vi "TEST_bench_Hyst_op_fxp_16_5.vi"(7 "N_hyst":i32) -> ()   [LabVIEW 2017]
uses:
  <vilib>/Platform/TimedLoop/XDataNode/timing_clust.ctl
  <vilib>/Platform/TimedLoop/XDataNode/nitl_modes.ctl
  <vilib>/Platform/TimedLoop/XDataNode/wakeup.ctl
  <vilib>/rvi/Emulation/niFpgaSctlEmulationGetInTimedLoop.vi
  <vilib>/rvi/Emulation/niFpgaEmulationReportErrorSimple.vi
  <vilib>/rvi/Emulation/niFpgaGetClockAttributes.vi
  <vilib>/rvi/Emulation/niFpgaCriticalErrorInLSC.vi
  <vilib>/rvi/Memory/Memory_Emulation/nirvimemoryFastEmulation.vi
  <vilib>/rvi/Memory/Memory_Emulation/nirvimemoryEmulation.vi
  <vilib>/rvi/Emulation/niFpgaEmulationIsFPGAContextNoSignature.vi
  <vilib>/rvi/DataTransferAndStorage/Container/Common/niFpgaContainerGetUniqueNameForEmu.vi
  <vilib>/rvi/Emulation/niFpgaProcessEmulError.vi
  <vilib>/rvi/errors/nirviReportUnexpectedCaseInternalError (U32).vi
  <vilib>/Platform/TimedLoop/XDataNode/XDataNode.xnode
  <vilib>/rvi/DataTransferAndStorage/Container/XNode/niFpgaContainer.xnode
  <vilib>/Platform/TimedLoop/XDataNode/XDNodeRunTimeDep.lvlib
panel:
  out "y_out_mem":fxp<+/-,16,5>[](array[numeric])
  out "S_of_ik (expected)":sgl[](array[numeric])
  out "H_of_uk":fxp<+/-,32,10>[](array[numeric])
  in  "uk":sgl[](array[numeric]) format="%#_13g"
  in  "numIter":i32
  in  "r_s":fxp<+/-,16,5>[](array[numeric])=[0.0, 0.82861328125, 1.8125, 2.8671875, 4.03173828125, 5.2001953125, 7.20166015625]
  in  "w_s":fxp<+/-,16,5>[](array[numeric])=[0.0, 0.0, 0.0, 0.0, 0.0, 0.0, 0.0]
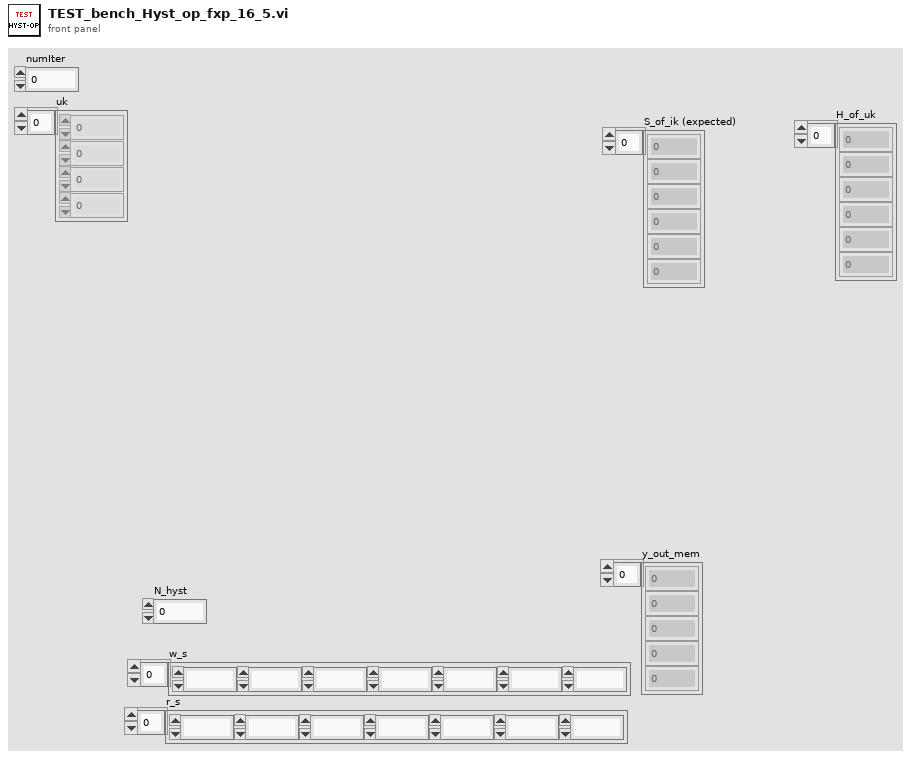
[diagram p1: front panel]
types:
  T1 = typedef "XDNodeRunTimeDep.lvlib/timing_clust.ctl" = cluster{"Expected End [f-1]":u64, "Actual End [f-1]":u64, "Finished Late? [f-1]":bool, "Expected End [i-1]":u64, "Actual End [i-1]":u64, "Finished Late? [i-1]":bool, "Expected Start [i]":u64, "Actual Start [i]":u64, "Expected Start [f]":u64, "Actual Start [f]":u64, "Source Name":string, "Structure Name":string, "Period":i64, "Deadline":i64, "Offset":i64, "Start":i64, "Priority":i32, "Timeout":i32, "Mode":T2, "Wakeup Reason":T3, "Error":errorcluster, "Source Type":string, "Secondary Source Type":string, "Global End Time":u64, "Global Start Time":u64, "Frame Duration":u64, "Iteration Duration":u64, "Assigned CPU":i32, "I/O Scan Engine Mode":u32}
  T2 = typedef "XDNodeRunTimeDep.lvlib/nitl_modes.ctl" = enum32{"No Change", "Process missed periods, maintain original phase", "Discard missed periods, maintain original phase", "Process missed periods, ignore original phase", "Discard missed periods, ignore original phase"}
  T3 = typedef "XDNodeRunTimeDep.lvlib/wakeup.ctl" = enum32{"Normal", "Aborted", "Asynchronous wakeup", "Timing source error", "Timed loop error", "Timeout"}
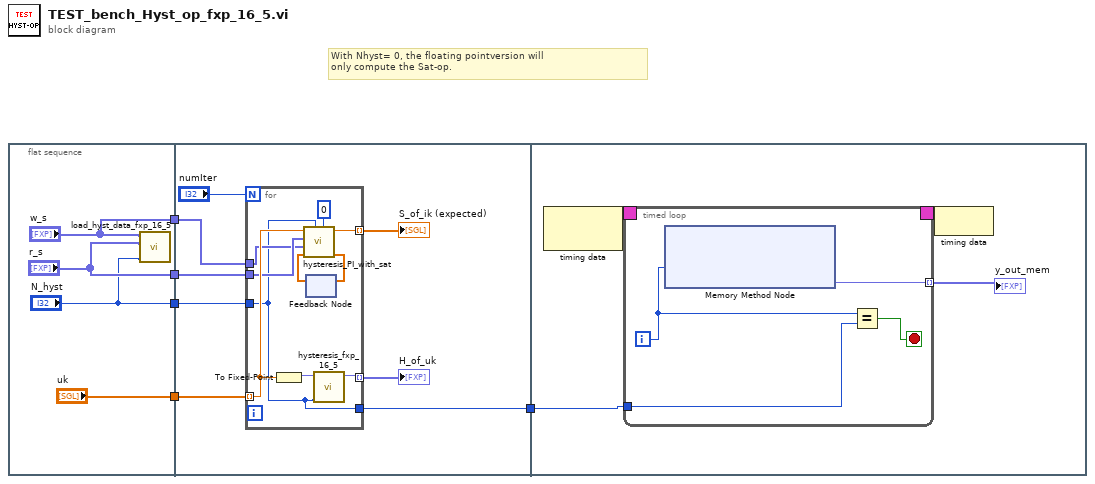
[diagram p0: block diagram]
diagram:
  # "With Nhyst= 0, the floating pointversion will\nonly compute the Sat-op."
  n1 = flat-sequence {
    tunnel: ["uk"] -> w5
    tunnel: ["w_s"] -> w4
    tunnel: ["r_s"] -> w3
    tunnel: ["N_hyst"] -> w2
    tunnel: w5 -> [w14]
    tunnel: w4 -> [w13]
    tunnel: w3 -> [w12]
    tunnel: w2 -> [w11]
    tunnel: [w10] -> w1
    tunnel: w1 -> [w28]
    frame #0 {
      n2 = call "load_hyst_data_fxp_16_5.vi"("N_hyst"="N_hyst", "r_s"="r_s", "w_s"="w_s") -> ()  [unwired: 9 in]
    }
    frame #1 {
      n3 = for {
        N: "numIter" -> [_]
        tunnel: [w25] -> w16 mode=indexing
        tunnel: w13 -> [w22]
        tunnel: w12 -> [w23]
        tunnel: [w27] -> w17 mode=indexing
        tunnel: w14 -> [w26] mode=indexing
        tunnel: w11 -> [w18]
        tunnel: [w18] -> w10
        n4 = To Fixed-Point(number=w26) -> (fixed-point=w24:fxp<+/-,16,5>)  [unwired: 1 in]
        n5 = feedback #1() -> (w20:sgl[])  [unwired: 1 in]
        n6 = call "hysteresis_PI_with_sat.vi"("N_sat"=0 ("N_hyst"), "N_hyst"=w18, "y_vec_in"=w20, "w_s"=w22, "r_s"=w23, "uk"=w26) -> ("y_vec_out"=w21:sgl[], "H_of_ik"=w27:sgl)  [unwired: 4 in]
        n7 = feedback-in #1(w21) -> ()
        n8 = call "hysteresis_fxp_16_5.vi"("N_hyst"=w18, "uk_in"=w24) -> ("Hinv(uk)"=w25:fxp<+/-,32,10>)  [unwired: 9 in]
      }
      "H_of_uk" <- w16
      "S_of_ik (expected)" <- w17
    }
    frame #2 {
      n9 = node-c288() -> (w31:T1)  [unwired: 1 in]
      n10 = timed-loop {
        timing: w31 -> [_]
        timing-out: [_] -> w30
        tunnel: [w35] -> w29 mode=indexing
        tunnel: w28 -> [w32]
        i -> [w33]
        stop <- w34 stop-if-true
        n11 = xnode ("Memory Method Node")("Address"=w33) -> ("Data"=w35:fxp<+/-,16,5>)  [unwired: 1 in, 1 out]
        n12 = Equal?(x=w33, y=w32) -> (x = y?=w34:bool)
      }
      "y_out_mem" <- w29
      n13 = node-c288(w30) -> ()
    }
  }
